vi "Find Opposite Point.vi"(7 "Circle Max Value":dbl, 10 "Circle Min Value":dbl, 11 "Position To invert":dbl) -> (3 "Opposite Point Out":dbl)   [LabVIEW 2023, in "SwerveDrive_ACT_ts.lvlib"]
uses:
  SwerveDrive_ACT_ts.lvlib
panel:
  out "Overflow":dbl
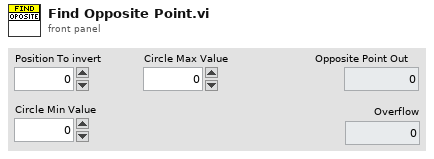
[diagram p1: front panel]
types:
  T1 = typedef "Dial_Compase heading unit circle CCW positive.ctl" = dbl
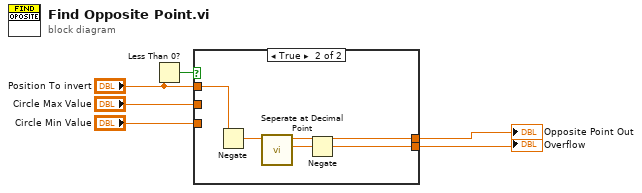
[diagram p0: block diagram]
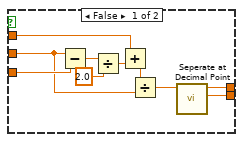
[diagram p2: hidden frame]
diagram:
  n1 = Less Than 0?(x="Position To invert") -> (x < 0?=w3:bool)
  n2 = case shown="True" w3 {
    tunnel: "Circle Min Value" -> [w16 _]
    tunnel: "Circle Max Value" -> [w11 _]
    tunnel: "Position To invert" -> [w10 w21]
    tunnel: [w7 w17] -> w2
    tunnel: [w8 w18] -> w1
    frame False {
      n3 = Subtract(x=w11, y=w16) -> (x-y=w15:dbl)
      n4 = Divide(x=w15, y=2.0) -> (x/y=w13:dbl)
      n5 = Add(x=w10, y=w13) -> (x+y=w12:dbl)
      n6 = Divide(x=w12, y=w11) -> (x/y=w9:dbl)
      n7 = call "Seperate at Decimal Point.vi"("Rotations"=w9) -> ("Rotations"=w7:dbl, "Angle"=w8:T1)  [unwired: 9 in]
    }
    frame True {
      n8 = Negate(x=w21) -> (-x=w20:dbl)
      n9 = call "Seperate at Decimal Point.vi"("Rotations"=w20) -> ("Rotations"=w19:dbl, "Angle"=w18:T1)  [unwired: 9 in]
      n10 = Negate(x=w19) -> (-x=w17:dbl)
    }
  }
  "Opposite Point Out" <- w1
  "Overflow" <- w2
